vi "ws_www template read file.vi"(6 "User":T1, 8 "error in (no error)":errorcluster, 11 "Template File (\"\")":string) -> (0 "error out":errorcluster, 3 "Page HTML":string)   [LabVIEW 2011]
uses:
  server/database/Users/User Record.ctl
  <userlib>/_OpenG.lib/file/file.llb/File Exists - Scalar__ogtk.vi
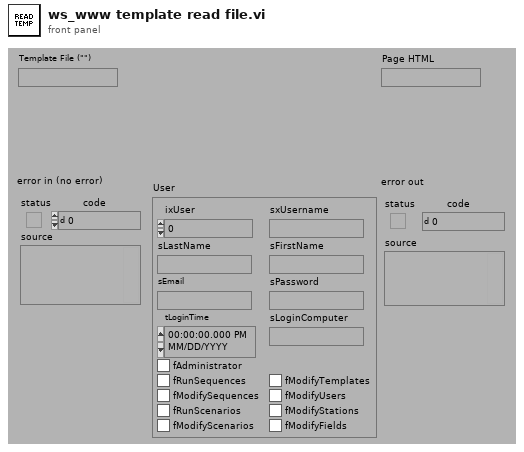
[diagram p1: front panel]
types:
  T1 = typedef "User Record.ctl" = cluster{"ixUser":i32, "sxUsername":string, "sLastName":string, "sFirstName":string, "sEmail":string, "sPassword":string, "tLoginTime":timestamp, "sLoginComputer":string, "fAdministrator":bool, "fRunSequences":bool, "fModifySequences":bool, "fRunScenarios":bool, "fModifyScenarios":bool, "fModifyTemplates":bool, "fModifyUsers":bool, "fModifyStations":bool, "fModifyFields":bool}
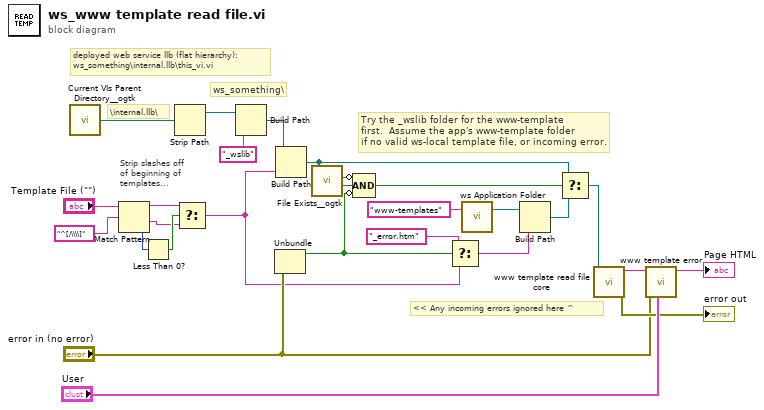
[diagram p0: block diagram]
diagram:
  # "Try the _wslib folder for the www-template\nfirst.  Assume the app's www-template folder\nif no valid ws-local template file, or incoming error."
  # "ws_something\\"
  # "\\internal.llb\\"
  # "deployed web service llb (flat hierarchy):\nws_something\\internal.llb\\this_vi.vi"
  # "Strip slashes off\nof beginning of\ntemplates..."
  # "<< Any incoming errors ignored here ^"
  n1 = call <userlib>:"Current VIs Parent Directory__ogtk.vi"() -> ("Parent Directory (+ Relative)"=w12:path)  [unwired: 5 in]
  n2 = Match Pattern(string="Template File (\"\")", regular expression="^[/\\\\]") -> (before substring=w24:string, after substring=w23:string, offset past match=w26:i32)  [unwired: 2 out]
  n3 = Less Than 0?(x=w26) -> (x < 0?=w25:bool)
  n4 = Strip Path(path=w12) -> (stripped path=w11:path)  [unwired: 1 out]
  n5 = Select(t=w24, s=w25, f=w23) -> (s? t:f=w8:string)
  n6 = Build Path(base path=w11, name or relative path="_wslib") -> (appended path=w9:path)
  n7 = Unbundle("error in (no error)") -> ("status"=w5:bool)  [unwired: 2 out]
  n8 = Build Path(base path=w9, name or relative path=w8) -> (appended path=w3:path)
  n9 = call-poly <userlib>:"File Exists__ogtk.vi"("file path"=w3) -> ("is directory"=w7:bool, "exists"=w6:bool)  [unwired: 6 in]
  n10 = Compound Arithmetic op=AND(invert w7, w6, invert w5) -> (w4:bool)
  n11 = Select(t="_error.htm" ("format string"), s=w5, f=w8) -> (s? t:f=w13:string)
  n12 = call "ws Application Folder.vi"("Relative Path (\"\" - Folder)"="www-templates" ("name or relative path")) -> ("Application Folder"=w14:path)  [unwired: 2 in]
  n13 = Build Path(base path=w14, name or relative path=w13) -> (appended path=w2:path)
  n14 = Select(t=w3, s=w4, f=w2) -> (s? t:f=w1:path)
  n15 = call "www template read file core.vi"("Path"=w1) -> ("error out"=→"error out":errorcluster, "File Content"=w17:string)  [unwired: 1 in, 8 out]
  n16 = call "www template error.vi"("User Information"="User", "error in (no error)"="error in (no error)", "Incoming Template HTML (\"\")"=w17) -> ("error.htm"=→"Page HTML":string)  [unwired: 8 out]
